vi "ScanBodyVideoInOptionConfig.vi"(11 "body":string="table.VideoInOptions[0].AlarmDayNightColorMode=0\r\ntable.VideoInOptions[0].AntiFlicker=0\r\ntable.VideoInOptions[0].AutoSyncPhase=false\r\ntable.VideoInOptions[0].Backlight=0\r\ntable.VideoInOptions[0].BacklightRegion[0]=3096\r\ntable.VideoInOptions[0].BacklightRegion[1]=3096\r\ntable.VideoInOptions[0].BacklightRegion[2]=5096\r\ntable.VideoInOptions[0].BacklightRegion[3]=5096\r\ntable.VideoInOptions[0].ColorTemperatureLevel=100\r\ntable.VideoInOptions[0].DayNightColor=1\r\ntable.VideoInOptions[0].DayNightSensitivity=2\r\ntable.VideoInOptions[0].DayNightSwitchDelay=6\r\ntable.VideoInOptions[0].DoubleExposure=0\r\ntable.VideoInOptions[0].DuskOptions.ExternalSyncPhase=125\r\ntable.VideoInOptions[0].ExposureIris=50\r\ntable.VideoInOptions[0].ExposureMode=0\r\ntable.VideoInOptions[0].ExposureSpeed=0\r\ntable.VideoInOptions[0].ExposureValue1=0\r\ntable.VideoInOptions[0].ExposureValue2=40\r\ntable.VideoInOptions[0].ExternalSync=0\r\ntable.VideoInOptions[0].ExternalSyncPhase=125\r\ntable.VideoInOptions[0].FlashControl.Mode=0\r\ntable.VideoInOptions[0].FlashControl.Pole=0\r\ntable.VideoInOptions[0].FlashControl.PreValue=40\r\ntable.VideoInOptions[0].FlashControl.Value=0\r\ntable.VideoInOptions[0].Flip=false\r\ntable.VideoInOptions[0].FocusMode=0\r\ntable.VideoInOptions[0].FocusRect[0]=0\r\ntable.VideoInOptions[0].FocusRect[1]=0\r\ntable.VideoInOptions[0].FocusRect[2]=8191\r\ntable.VideoInOptions[0].FocusRect[3]=8191\r\ntable.VideoInOptions[0].Gain=50\r\ntable.VideoInOptions[0].GainAuto=true\r\ntable.VideoInOptions[0].GainBlue=50\r\ntable.VideoInOptions[0].GainGreen=50\r\ntable.VideoInOptions[0].GainMax=50\r\ntable.VideoInOptions[0].GainMin=0\r\ntable.VideoInOptions[0].GainRed=50\r\ntable.VideoInOptions[0].GlareInhibition=0\r\ntable.VideoInOptions[0].InfraRed=false\r\ntable.VideoInOptions[0].InfraRedLevel=0\r\ntable.VideoInOptions[0].IrisAuto=true\r\ntable.VideoInOptions[0].IrisAutoSensitivity=50\r\ntable.VideoInOptions[0].Mirror=true\r\ntable.VideoInOptions[0].NightOptions.AlarmDayNightColorMode=0\r\ntable.VideoInOptions[0].NightOptions.AntiFlicker=0\r\ntable.VideoInOptions[0].NightOptions.Backlight=0\r\ntable.VideoInOptions[0].NightOptions.BacklightRegion[0]=3096\r\ntable.VideoInOptions[0].NightOptions.BacklightRegion[1]=3096\r\ntable.VideoInOptions[0].NightOptions.BacklightRegion[2]=5096\r\ntable.VideoInOptions[0].NightOptions.BacklightRegion[3]=5096\r\ntable.VideoInOptions[0].NightOptions.BrightnessThreshold=50\r\ntable.VideoInOptions[0].NightOptions.DayNightColor=1\r\ntable.VideoInOptions[0].NightOptions.DayNightSensitivity=2\r\ntable.VideoInOptions[0].NightOptions.DayNightSwitchDelay=6\r\ntable.VideoInOptions[0].NightOptions.ExposureIris=50\r\ntable.VideoInOptions[0].NightOptions.ExposureMode=0\r\ntable.VideoInOptions[0].NightOptions.ExposureSpeed=0\r\ntable.VideoInOptions[0].NightOptions.ExposureValue1=0\r\ntable.VideoInOptions[0].NightOptions.ExposureValue2=40\r\ntable.VideoInOptions[0].NightOptions.ExternalSyncPhase=125\r\ntable.VideoInOptions[0].NightOptions.Flip=false\r\ntable.VideoInOptions[0].NightOptions.Gain=50\r\ntable.VideoInOptions[0].NightOptions.GainAuto=true\r\ntable.VideoInOptions[0].NightOptions.GainBlue=50\r\ntable.VideoInOptions[0].NightOptions.GainGreen=50\r\ntable.VideoInOptions[0].NightOptions.GainMax=50\r\ntable.VideoInOptions[0].NightOptions.GainMin=0\r\ntable.VideoInOptions[0].NightOptions.GainRed=50\r\ntable.VideoInOptions[0].NightOptions.GlareInhibition=0\r\ntable.VideoInOptions[0].NightOptions.InfraRed=false\r\ntable.VideoInOptions[0].NightOptions.InfraRedLevel=0\r\ntable.VideoInOptions[0].NightOptions.IrisAuto=true\r\ntable.VideoInOptions[0].NightOptions.IrisAutoSensitivity=50\r\ntable.VideoInOptions[0].NightOptions.Mirror=true\r\ntable.VideoInOptions[0].NightOptions.Profile=3\r\ntable.VideoInOptions[0].NightOptions.ReferenceLevel=50\r\ntable.VideoInOptions[0].NightOptions.Rotate90=0\r\ntable.VideoInOptions[0].NightOptions.SunriseHour=0\r\ntable.VideoInOptions[0].NightOptions.SunriseMinute=0\r\ntable.VideoInOptions[0].NightOptions.SunriseSecond=0\r\ntable.VideoInOptions[0].NightOptions.SunsetHour=24\r\ntable.VideoInOptions[0].NightOptions.SunsetMinute=0\r\ntable.VideoInOptions[0].NightOptions.SunsetSecond=0\r\ntable.VideoInOptions[0].NightOptions.SwitchMode=0\r\ntable.VideoInOptions[0].NightOptions.TemporaryConfigs.AntiFlicker=0\r\ntable.VideoInOptions[0].NightOptions.TemporaryConfigs.ExposureMode=0\r\ntable.VideoInOptions[0].NightOptions.TemporaryConfigs.ExposureValue1=0.100000\r\ntable.VideoInOptions[0].NightOptions.TemporaryConfigs.ExposureValue2=80\r\ntable.VideoInOptions[0].NightOptions.TemporaryConfigs.GainMax=50\r\ntable.VideoInOptions[0].NightOptions.TemporaryConfigs.GainMin=10\r\ntable.VideoInOptions[0].NightOptions.WhiteBalance=Auto\r\ntable.VideoInOptions[0].NightOptions.WhiteBalanceDatumRect[0]=0\r\ntable.VideoInOptions[0].NightOptions.WhiteBalanceDatumRect[1]=0\r\ntable.VideoInOptions[0].NightOptions.WhiteBalanceDatumRect[2]=1000\r\ntable.VideoInOptions[0].NightOptions.WhiteBalanceDatumRect[3]=1000\r\ntable.VideoInOptions[0].NightOptions.WideDynamicRange=0\r\ntable.VideoInOptions[0].NightOptions.WideDynamicRangeMode=0\r\ntable.VideoInOptions[0].NormalOptions.AlarmDayNightColorMode=0\r\ntable.VideoInOptions[0].NormalOptions.AntiFlicker=0\r\ntable.VideoInOptions[0].NormalOptions.Backlight=0\r\ntable.VideoInOptions[0].NormalOptions.BacklightRegion[0]=3096\r\ntable.VideoInOptions[0].NormalOptions.BacklightRegion[1]=3096\r\ntable.VideoInOptions[0].NormalOptions.BacklightRegion[2]=5096\r\ntable.VideoInOptions[0].NormalOptions.BacklightRegion[3]=5096\r\ntable.VideoInOptions[0].NormalOptions.BrightnessThreshold=50\r\ntable.VideoInOptions[0].NormalOptions.DayNightColor=1\r\ntable.VideoInOptions[0].NormalOptions.DayNightSensitivity=2\r\ntable.VideoInOptions[0].NormalOptions.DayNightSwitchDelay=6\r\ntable.VideoInOptions[0].NormalOptions.ExposureIris=50\r\ntable.VideoInOptions[0].NormalOptions.ExposureMode=0\r\ntable.VideoInOptions[0].NormalOptions.ExposureSpeed=0\r\ntable.VideoInOptions[0].NormalOptions.ExposureValue1=0\r\ntable.VideoInOptions[0].NormalOptions.ExposureValue2=40\r\ntable.VideoInOptions[0].NormalOptions.ExternalSyncPhase=125\r\ntable.VideoInOptions[0].NormalOptions.Flip=false\r\ntable.VideoInOptions[0].NormalOptions.Gain=50\r\ntable.VideoInOptions[0].NormalOptions.GainAuto=true\r\ntable.VideoInOptions[0].NormalOptions.GainBlue=50\r\ntable.VideoInOptions[0].NormalOptions.GainGreen=50\r\ntable.VideoInOptions[0].NormalOptions.GainMax=50\r\ntable.VideoInOptions[0].NormalOptions.GainMin=0\r\ntable.VideoInOptions[0].NormalOptions.GainRed=50\r\ntable.VideoInOptions[0].NormalOptions.GlareInhibition=0\r\ntable.VideoInOptions[0].NormalOptions.InfraRed=false\r\ntable.VideoInOptions[0].NormalOptions.InfraRedLevel=0\r\ntable.VideoInOptions[0].NormalOptions.IrisAuto=true\r\ntable.VideoInOptions[0].NormalOptions.IrisAutoSensitivity=50\r\ntable.VideoInOptions[0].NormalOptions.Mirror=true\r\ntable.VideoInOptions[0].NormalOptions.Profile=0\r\ntable.VideoInOptions[0].NormalOptions.ReferenceLevel=50\r\ntable.VideoInOptions[0].NormalOptions.Rotate90=0\r\ntable.VideoInOptions[0].NormalOptions.SunriseHour=0\r\ntable.VideoInOptions[0].NormalOptions.SunriseMinute=0\r\ntable.VideoInOptions[0].NormalOptions.SunriseSecond=0\r\ntable.VideoInOptions[0].NormalOptions.SunsetHour=23\r\ntable.VideoInOptions[0].NormalOptions.SunsetMinute=59\r\ntable.VideoInOptions[0].NormalOptions.SunsetSecond=59\r\ntable.VideoInOptions[0].NormalOptions.SwitchMode=0\r\ntable.VideoInOptions[0].NormalOptions.TemporaryConfigs.AntiFlicker=0\r\ntable.VideoInOptions[0].NormalOptions.TemporaryConfigs.ExposureMode=0\r\ntable.VideoInOptions[0].NormalOptions.TemporaryConfigs.ExposureValue1=0.100000\r\ntable.VideoInOptions[0].NormalOptions.TemporaryConfigs.ExposureValue2=80\r\ntable.VideoInOptions[0].NormalOptions.TemporaryConfigs.GainMax=50\r\ntable.VideoInOptions[0].NormalOptions.TemporaryConfigs.GainMin=10\r\ntable.VideoInOptions[0].NormalOptions.WhiteBalance=Auto\r\ntable.VideoInOptions[0].NormalOptions.WhiteBalanceDatumRect[0]=0\r\ntable.VideoInOptions[0].NormalOptions.WhiteBalanceDatumRect[1]=0\r\ntable.VideoInOptions[0].NormalOptions.WhiteBalanceDatumRect[2]=1000\r\ntable.VideoInOptions[0].NormalOptions.WhiteBalanceDatumRect[3]=1000\r\ntable.VideoInOptions[0].NormalOptions.WideDynamicRange=0\r\ntable.VideoInOptions[0].NormalOptions.WideDynamicRangeMode=0\r\ntable.VideoInOptions[0].ReferenceLevel=50\r\ntable.VideoInOptions[0].ReferenceLevelEnable=false\r\ntable.VideoInOptions[0].Rotate90=0\r\ntable.VideoInOptions[0].SignalFormat=Inside\r\ntable.VideoInOptions[0].Snapshot.ColorTemperatureLevel=50\r\ntable.VideoInOptions[0].Snapshot.ExposureSpeed=0\r\ntable.VideoInOptions[0].Snapshot.ExposureValue1=0\r\ntable.VideoInOptions[0].Snapshot.ExposureValue2=40\r\ntable.VideoInOptions[0].Snapshot.Gain=50\r\ntable.VideoInOptions[0].Snapshot.GainAuto=true\r\ntable.VideoInOptions[0].Snapshot.GainBlue=50\r\ntable.VideoInOptions[0].Snapshot.GainGreen=50\r\ntable.VideoInOptions[0].Snapshot.GainRed=50\r\ntable.VideoInOptions[0].Snapshot.WhiteBalance=Disable\r\ntable.VideoInOptions[0].TemporaryConfigs.AntiFlicker=0\r\ntable.VideoInOptions[0].TemporaryConfigs.ExposureMode=0\r\ntable.VideoInOptions[0].TemporaryConfigs.ExposureValue1=0.100000\r\ntable.VideoInOptions[0].TemporaryConfigs.ExposureValue2=80\r\ntable.VideoInOptions[0].TemporaryConfigs.GainMax=50\r\ntable.VideoInOptions[0].TemporaryConfigs.GainMin=10\r\ntable.VideoInOptions[0].WhiteBalance=Auto\r\ntable.VideoInOptions[0].WhiteBalanceDatumRect[0]=0\r\ntable.VideoInOptions[0].WhiteBalanceDatumRect[1]=0\r\ntable.VideoInOptions[0].WhiteBalanceDatumRect[2]=1000\r\ntable.VideoInOptions[0].WhiteBalanceDatumRect[3]=1000\r\ntable.VideoInOptions[0].WideDynamicRange=0\r\ntable.VideoInOptions[0].WideDynamicRangeMode=0\r\n") -> (3 "array type (2D Dbl)":string[][](array[string]))   [LabVIEW 2016]
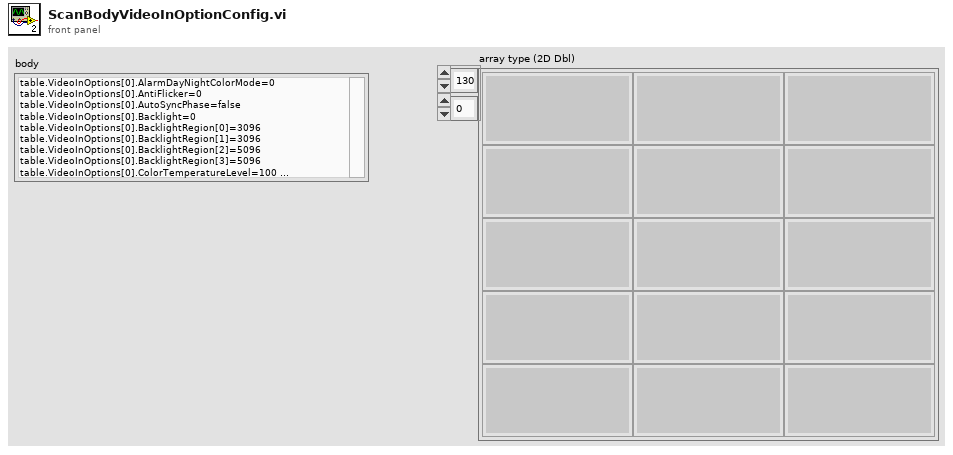
[diagram p1: front panel]
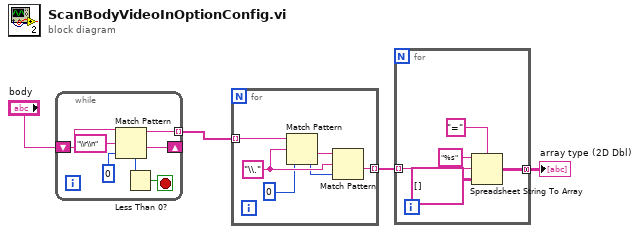
[diagram p0: block diagram]
diagram:
  n1 = while {
    tunnel: [w9] -> w2 mode=indexing
    shift-right: [w7] -> _
    shift-left: "body" -> [w6]
    stop <- w8 stop-if-true
    n2 = Match Pattern(string=w6, regular expression="\\r\\n", offset (0)=0 ("offset past match")) -> (before substring=w9:string, after substring=w7:string, offset past match=w10:i32)  [unwired: 1 out]
    n3 = Less Than 0?(x=w10) -> (x < 0?=w8:bool)
  }
  n4 = for {
    tunnel: w2 -> [w14] mode=indexing
    tunnel: [w13] -> w4 mode=indexing
    w16 = "\\." ("regular expression")
    n5 = Match Pattern(string=w14, regular expression=w16, offset (0)=0 ("offset past match")) -> (after substring=w17:string, offset past match=w15:i32)  [unwired: 2 out]
    n6 = Match Pattern(string=w17, regular expression=w16, offset (0)=w15) -> (after substring=w13:string)  [unwired: 3 out]
  }
  n7 = for {
    tunnel: w4 -> [w19] mode=indexing
    tunnel: [w18] -> w3 mode=concatenating
    n8 = Spreadsheet String To Array(delimiter (Tab)="=", format string="%s", spreadsheet string=w19, array type (2D Dbl)=string[][] []) -> (array=w18:string[][])
  }
  "array type (2D Dbl)" <- w3
